vi "Type Specialization Structure.vi"   [LabVIEW 2017]
doc: "Attempts to compile each of its frames in order and accepts the first one that has no syntax eror. Defaults to the last frame if all frames have suntax errors. Use this structure to build complex malleable VIs (.vim files) that can behave differently for different input types.\n\n \n\nThis structure is not a public LabVIEW feature. It is experimental and should not be edited, copied, or used in other VIs without conducting extensive testing."
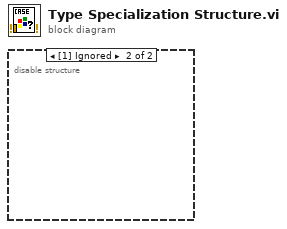
[diagram p0: block diagram]
diagram:
  n1 = disable-structure shown="[1] Ignored" {
    frame Enabled {
    }
    frame Disabled {
    }
  }
